vi "UI Interlocks.vi"(7 "FP Refs":T1, 8 "error in (no error)":errorcluster, 9 "Menu Ref":refnum<k9>, 10 "VI Selected":i32, 11 "New Item Data":refnum<class "Item.lvclass">[](array[class])) -> (0 "error out":errorcluster)   [LabVIEW 2020, in "VI Properties Editor.lvlib"]
doc: "Enables or disables several menu items and buttons depending on the state of the system."
uses:
  VI Properties Editor.lvlib
  Classes/Item/Item.lvclass
  Classes/VI/VI.lvclass
  CTLs/Main References.ctl
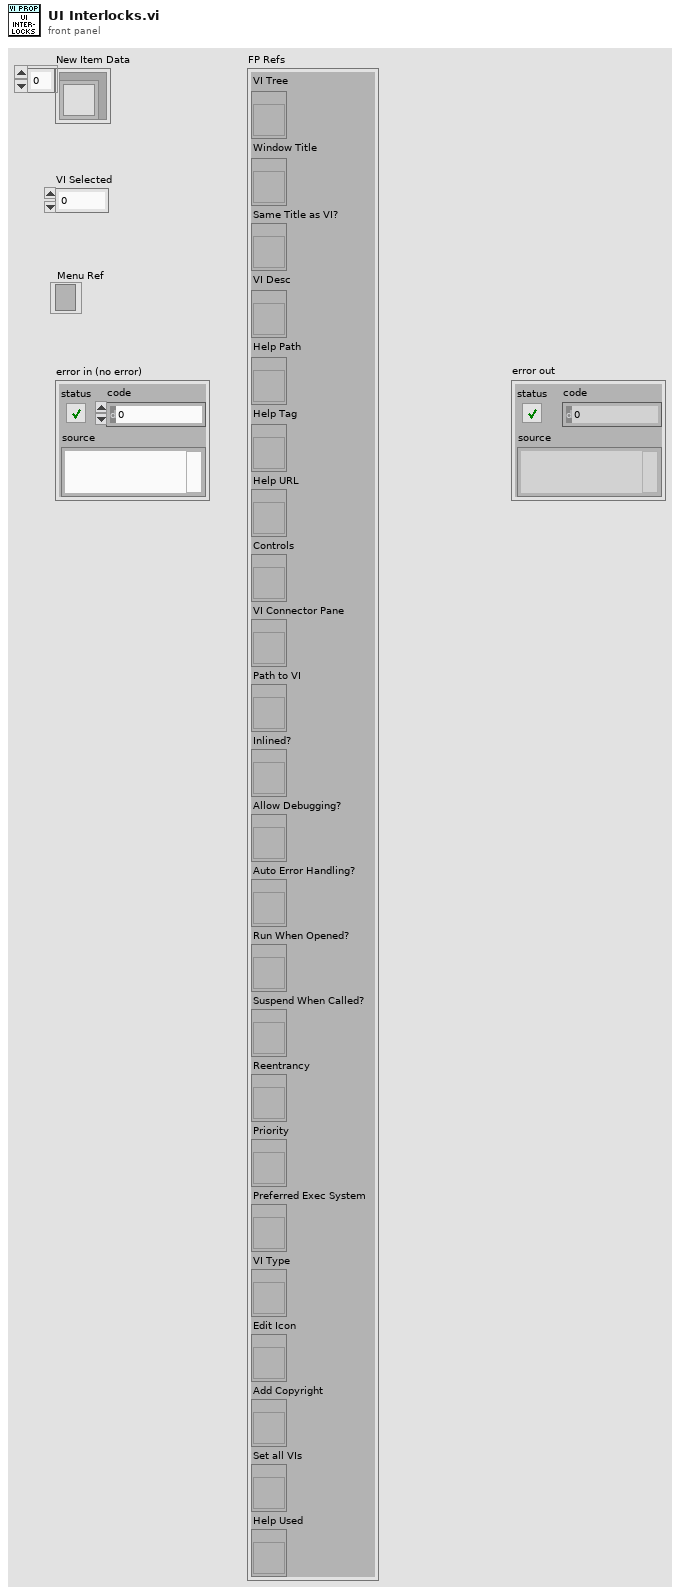
[diagram p1: front panel]
types:
  T1 = typedef "VI Properties Editor.lvlib/Main References.ctl" = cluster{"VI Tree":refnum<vi>, "Window Title":refnum<vi>, "Same Title as VI?":refnum<vi>, "VI Desc":refnum<vi>, "Help Path":refnum<vi>, "Help Tag":refnum<vi>, "Help URL":refnum<vi>, "Controls":refnum<vi>, "VI Connector Pane":refnum<vi>, "Path to VI":refnum<vi>, "Inlined?":refnum<vi>, "Allow Debugging?":refnum<vi>, "Auto Error Handling?":refnum<vi>, "Run When Opened?":refnum<vi>, "Suspend When Called?":refnum<vi>, "Reentrancy":refnum<vi>, "Priority":refnum<vi>, "Preferred Exec System":refnum<vi>, "VI Type":refnum<vi>, "Edit Icon":refnum<vi>, "Add Copyright":refnum<vi>, "Set all VIs":refnum<vi>, "Help Used":refnum<vi>}
  T2 = enum32{"invalid VI type", "Standard VI", "Control VI", "Global VI", "Polymorphic VI", "Configuration VI", "SubSystem", "Facade VI", "Method VI", "Statechart Diagram VI"}
  T3 = enum8{"Enabled", "Disabled", "Disabled and Grayed Out"}
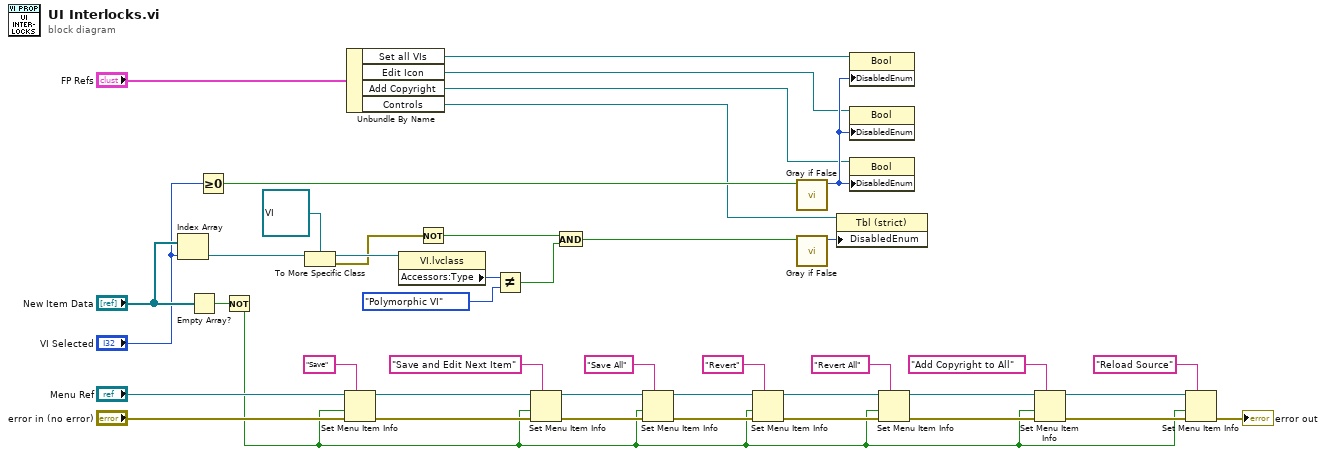
[diagram p0: block diagram]
diagram:
  n1 = Index Array(array="New Item Data", index="VI Selected") -> (element=w16:refnum<class "Item.lvclass">)
  n2 = Empty Array?(array="New Item Data") -> (empty?=w40:bool)
  n3 = Greater Or Equal To 0?(x="VI Selected") -> (x >= 0?=w22:bool)
  n4 = Not(x=w40) -> (.not. x?=w1:bool)
  n5 = To More Specific Class(target class=refnum<class "VI.lvclass"> refnum ("VI Properties Editor.lvlib:VI.lvclass"), reference=w16) -> (specific class reference=w20:refnum<class "VI.lvclass">, error out=w9:errorcluster)  [unwired: 1 in]
  n6 = Set Menu Item Info(7:"Save" ("item tag"), 8:"error in (no error)", 9:w1, 11:"Menu Ref") -> (0:w36:errorcluster, 3:w37:refnum<k9>)  [unwired: 3 in]
  n7 = Unbundle By Name("FP Refs") -> ("Set all VIs"=w14:refnum<vi>, "Edit Icon"=w12:refnum<vi>, "Add Copyright"=w11:refnum<vi>, "Controls"=w10:refnum<vi>)
  n8 = property class="VI.lvclass"(reference=w20) -> ("Accessors:Type"=w19:T2)  [unwired: 1 in, 2 out]
  n9 = Not(x=w9) -> (.not. x?=w8:bool)
  n10 = Not Equal?(x=w19, y=T2."Polymorphic VI" ("x")) -> (x != y?=w7:bool)
  n11 = Set Menu Item Info(7:"Save and Edit Next Item" ("item tag"), 8:w36, 9:w1, 11:w37) -> (0:w34:errorcluster, 3:w35:refnum<k9>)  [unwired: 3 in]
  n12 = And(x=w8, y=w7) -> (x .and. y?=w6:bool)
  n13 = Set Menu Item Info(7:"Save All" ("item tag"), 8:w34, 9:w1, 11:w35) -> (0:w31:errorcluster, 3:w32:refnum<k9>)  [unwired: 3 in]
  n14 = Set Menu Item Info(7:"Revert" ("item tag"), 8:w31, 9:w1, 11:w32) -> (0:w28:errorcluster, 3:w29:refnum<k9>)  [unwired: 3 in]
  n15 = call "Gray if False.vi"("Grayed Out?"=w22) -> ("Enabled State"=w13:T3)  [unwired: 10 in]
  n16 = call "Gray if False.vi"("Grayed Out?"=w6) -> ("Enabled State"=w23:T3)  [unwired: 10 in]
  n17 = property on="Property Node" class="Tbl (strict)"(reference=w10, "DisabledEnum"=w23) -> ()  [unwired: 1 in, 2 out]
  n18 = property on="Property Node" class="Bool"(reference=w14, "DisabledEnum"=w13) -> ()  [unwired: 1 in, 2 out]
  n19 = property on="Property Node" class="Bool"(reference=w12, "DisabledEnum"=w13) -> ()  [unwired: 1 in, 2 out]
  n20 = property on="Property Node" class="Bool"(reference=w11, "DisabledEnum"=w13) -> ()  [unwired: 1 in, 2 out]
  n21 = Set Menu Item Info(7:"Revert All" ("item tag"), 8:w28, 9:w1, 11:w29) -> (0:w26:errorcluster, 3:w25:refnum<k9>)  [unwired: 3 in]
  n22 = Set Menu Item Info(7:"Add Copyright to All" ("item tag"), 8:w26, 9:w1, 11:w25) -> (0:w2:errorcluster, 3:w3:refnum<k9>)  [unwired: 3 in]
  n23 = Set Menu Item Info(7:"Reload Source" ("item tag"), 8:w2, 9:w1, 11:w3) -> (0:→"error out":errorcluster)  [unwired: 3 in, 1 out]
